vi "Abort.vi"(0 "Notifier Name":string, 11 "Error In":errorcluster) -> (4 "Notifier Name DUP":string, 6 "Running?":bool, 10 "Image Ref":T1, 15 "Error Out":errorcluster)   [LabVIEW 2020]
uses:
  <vilib>/vision/Image Controls.llb/IMAQ Image.ctl
  Hardware Configuration/Hardware Configuration Controls/Company.ctl
  Hamamatsu/Orca Flash/Orca Flash Controls/Orca Flash Actions.ctl
  IDS/IDS Controls/IDS Actions.ctl
  Photometrics/Prime BSI/R Cubed SITK/Prime BSI R3 Controls/Prime R3 Actions.ctl
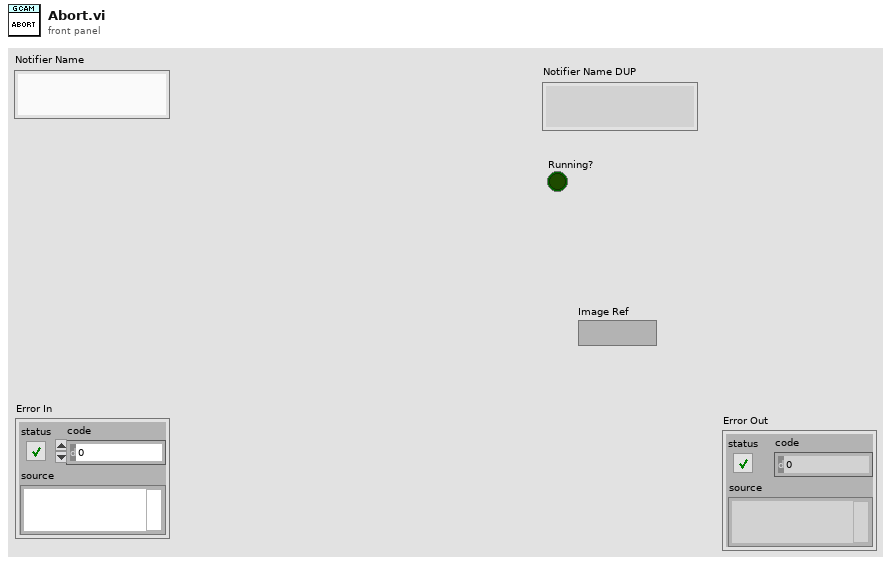
[diagram p1: front panel]
types:
  T1 = typedef "IMAQ Image.ctl" = refnum<image>
  T2 = typedef "Company.ctl" = enum16{"AA Opto Electronic", "ASI", "Coherent", "Creset Optics", "CVI", "DAQmx", "Hamamatsu", "IDS", "Mad City Labs", "Marzhauser", "Measurement Computing", "MPB Com", "Olympus", "Photometrics", "PI", "Prior", "Thorlabs"}
  T3 = typedef "Orca Flash Actions.ctl" = enum16{"Idle", "Preview", "Record", "Record Settings", "Set Param", "Get Param", "Set ROI", "Get ROI", "Trigger Source", "Trigger Type", "Progessive Mode", "Area Mode", "Status", "Quit"}
  T4 = typedef "IDS Actions.ctl" = enum16{"Error Check", "Initialize", "Preview", "Record", "Abort", "Record Settings", "Set Parameter", "Get Parameter", "Set ROI", "Get ROI", "Status", "Quit"}
  T5 = typedef "Prime R3 Actions.ctl" = enum16{"Error Check", "Initialize", "Preview", "Record", "Abort", "Record Settings", "Set Parameter", "Get Parameter", "Set ROI", "Get ROI", "Status", "Set Trigger", "Quit"}
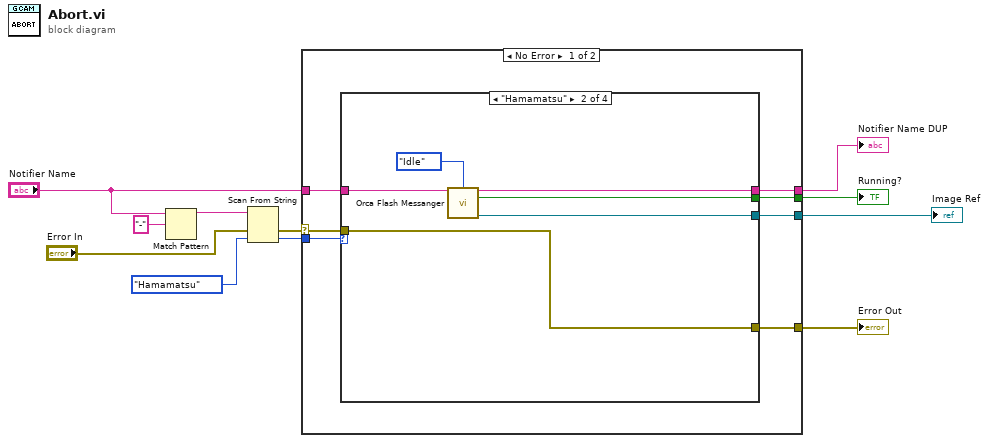
[diagram p0: block diagram]
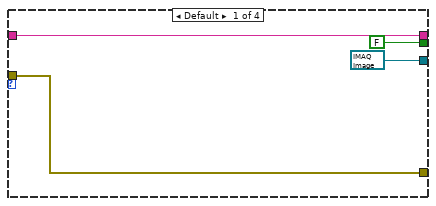
[diagram p2: hidden frame]
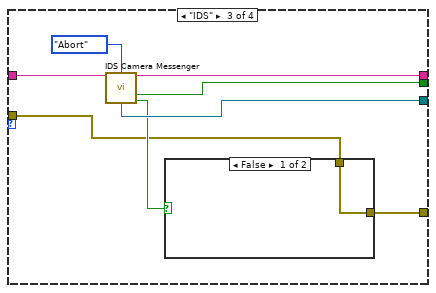
[diagram p3: hidden frame]
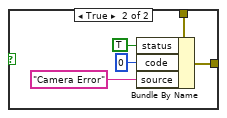
[diagram p4: hidden frame]
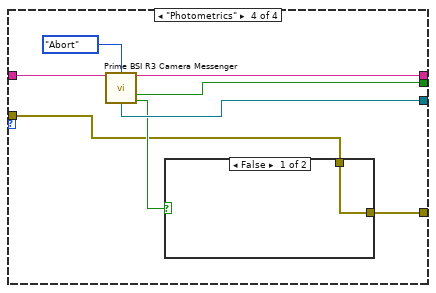
[diagram p5: hidden frame]
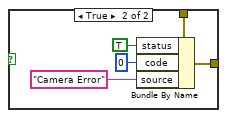
[diagram p6: hidden frame]
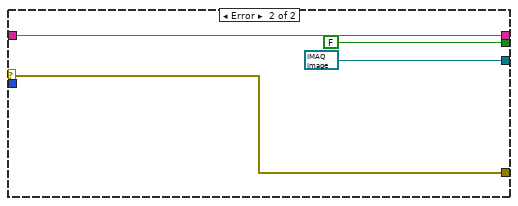
[diagram p7: hidden frame]
diagram:
  n1 = Match Pattern(string="Notifier Name", regular expression="-") -> (before substring=w9:string)  [unwired: 1 in, 3 out]
  n2 = Scan From String(input string=w9, error in="Error In", default 1=Company."Hamamatsu" ("Company")) -> (error out=w5:errorcluster, output 1=w8:T2)  [unwired: 2 in, 2 out]
  n3 = case shown="No Error" w5 {
    selector: w5 -> [w14 w59]
    tunnel: w8 -> [w18 _]
    tunnel: "Notifier Name" -> [w17 w60]
    tunnel: [w16 T1 refnum ("Image Ref")] -> w3
    tunnel: [w15 FALSE ("Running?")] -> w4
    tunnel: [w13 w60] -> w2
    tunnel: [w12 w59] -> w1
    frame No Error {
      n4 = case shown="\"Hamamatsu\"" w18 {
        tunnel: w17 -> [w22 w28 w36 w50]
        tunnel: [T1 refnum ("Image Ref") w26 w34 w48] -> w16
        tunnel: [FALSE ("Running?") w25 w33 w47] -> w15
        tunnel: w14 -> [w21 w23 w30 w45]
        tunnel: [w22 w24 w35 w49] -> w13
        tunnel: [w21 w23 w29 w44] -> w12
        frame Default {
        }
        frame "Hamamatsu" {
          n5 = call "Orca Flash Messanger.vi"("Notifier Name"=w28, "Camera Actions"=Orca_Flash_Actions."Idle") -> ("Notifier Name Dup"=w24:string, "Running?"=w25:bool, "Image Ref"=w26:T1)  [unwired: 9 in, 2 out]
        }
        frame "IDS" {
          n6 = call "IDS Camera Messenger.vi"("Notifier Name"=w36, "IDS Actions"=IDS_Actions."Abort") -> ("Notifier Name (Dup)"=w35:string, "Running?"=w33:bool, "Image Ref"=w34:T1, "Error?"=w31:bool)  [unwired: 8 in, 2 out]
          n7 = case shown="False" w31 {
            tunnel: w30 -> [w37 w42]
            tunnel: [w37 w41] -> w29
            frame False {
            }
            frame True {
              n8 = Bundle By Name(cluster=w42, "status"=TRUE, "code"=0, "source"="Camera Error") -> (w41:errorcluster)
            }
          }
        }
        frame "Photometrics" {
          n9 = call "Prime BSI R3 Camera Messenger.vi"("Notifier Name"=w50, "Prime Actions"=Prime_R3_Actions."Abort") -> ("Notifier Name (Dup)"=w49:string, "Running?"=w47:bool, "Image Ref"=w48:T1, "Error?"=w46:bool)  [unwired: 8 in, 2 out]
          n10 = case shown="False" w46 {
            tunnel: w45 -> [w51 w56]
            tunnel: [w51 w55] -> w44
            frame False {
            }
            frame True {
              n11 = Bundle By Name(cluster=w56, "status"=TRUE, "code"=0, "source"="Camera Error") -> (w55:errorcluster)
            }
          }
        }
      }
    }
    frame Error {
    }
  }
  "Error Out" <- w1
  "Notifier Name DUP" <- w2
  "Image Ref" <- w3
  "Running?" <- w4
